vi "AB_860_900_Project_SourceItems.vi"(5 "Provider Item":T1, 7 "action":T2, 8 "error in (no error)":errorcluster, 10 "oldBuildObject":T1, 11 "buildObject":T1) -> (0 "error out":errorcluster, 3 "buildObject out":T1)   [LabVIEW 2020]
doc: "Reads and writes the data to the object property bag."
uses:
  <resource>/Framework/Providers/API/ItemRef.ctl
  <vilib>/AppBuilder/RW_Project/AB_RW_Project_PropBag_ArrayAction.ctl
  <vilib>/AppBuilder/RW_Project/AB_RW_Project_PropBag_Action.ctl
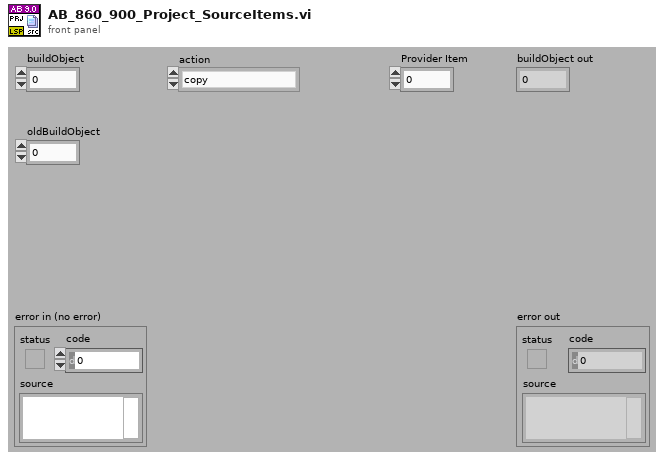
[diagram p1: front panel]
types:
  T1 = typedef "ItemRef.ctl" = u64
  T2 = typedef "AB_RW_Project_PropBag_ArrayAction.ctl" = enum16{"copy", "saveForPrevious", "loadFromPrevious", "clear"}
  T3 = typedef "AB_RW_Project_PropBag_Action.ctl" = enum16{"read", "write", "clear", "readPrevious", "writePrevious", "clearPrevious"}
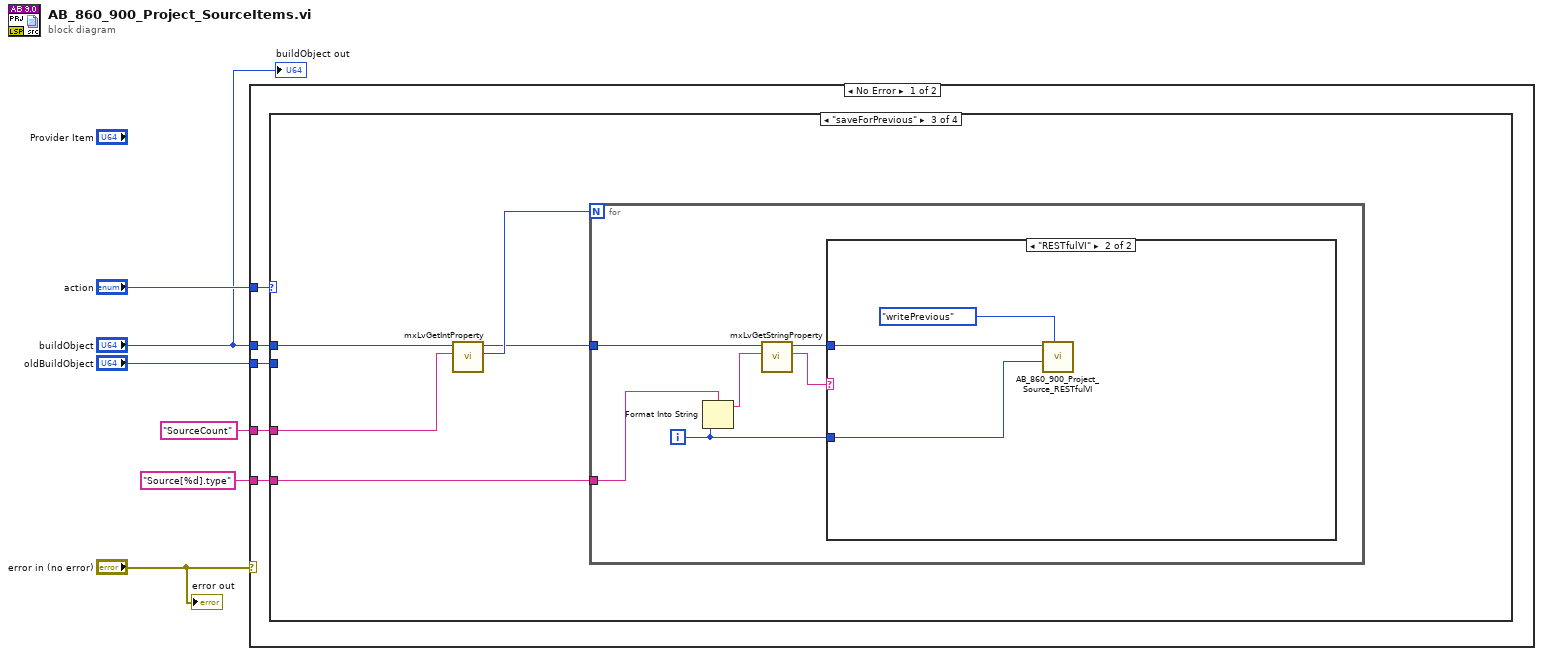
[diagram p0: block diagram]
diagram:
  n1 = case shown="No Error" "error in (no error)" {
    tunnel: "action" -> [w11 _]
    tunnel: "buildObject" -> [w10 _]
    tunnel: "SourceCount" -> [w9 _]
    tunnel: "Source[%d].type" -> [w8 _]
    tunnel: "oldBuildObject" -> [w7 _]
    frame No Error {
      n2 = case shown="\"saveForPrevious\"" w11 {
        tunnel: w10 -> [_ _ w13 _]
        tunnel: w9 -> [_ _ w14 _]
        tunnel: w8 -> [_ _ w12 _]
        tunnel: w7 -> [_ _ _ _]
        frame "copy" {
        }
        frame "loadFromPrevious" {
        }
        frame "saveForPrevious" {
          n3 = call <resource>:"mxLvGetIntProperty.vi"("Tag"=w14, "Item"=w13) -> ("Value"=w16:i32, "Item"=w15:T1)  [unwired: 1 in, 7 out]
          n4 = for {
            N: w16 -> [_]
            tunnel: w12 -> [w22]
            tunnel: w15 -> [w20]
            i -> [w21]
            n5 = Format Into String(format string=w22, w21) -> (resulting string=w19:string)  [unwired: 2 in, 1 out]
            n6 = call <resource>:"mxLvGetStringProperty.vi"("Tag"=w19, "Item"=w20) -> ("Value"=w18:string, "Item"=w17:T1)  [unwired: 1 in, 7 out]
            n7 = case shown="\"RESTfulVI\"" w18 {
              tunnel: w17 -> [_ w25]
              tunnel: w21 -> [_ w23]
              frame Default {
              }
              frame "RESTfulVI" {
                n8 = call <vilib>:"AB_860_900_Project_Source_RESTfulVI.vi"("action"=AB_RW_Project_PropBag_Action."writePrevious", "index in"=w23, "buildObject"=w25) -> ()  [unwired: 5 in, 4 out]
              }
            }
          }
        }
        frame "clear" {
        }
      }
    }
    frame Error {
    }
  }
  "error out" <- "error in (no error)"
  "buildObject out" <- "buildObject"
